vi "Logger.Stats.ListFiles.vi"(8 "error in (no error)":errorcluster) -> (0 "error out":errorcluster, 2 "Files":path[](array[path]))   [LabVIEW 2016]
uses:
  Global/ApplicationGlobal.vi
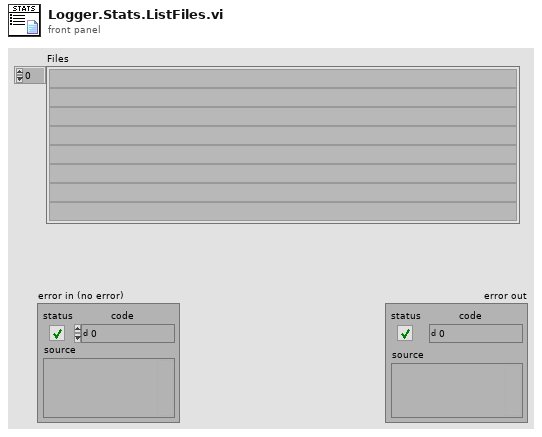
[diagram p1: front panel]
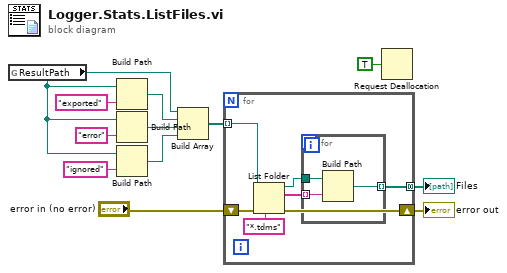
[diagram p0: block diagram]
diagram:
  n1 = global read "ApplicationGlobal.vi" "ResultPath"() -> (w5:path)
  n2 = Build Path(base path=w5, name or relative path="exported") -> (appended path=w9:path)
  n3 = Build Path(base path=w5, name or relative path="error") -> (appended path=w6:path)
  n4 = Build Path(base path=w5, name or relative path="ignored") -> (appended path=w8:path)
  n5 = Build Array(w5, w9, w6, w8) -> (w7:path[])
  n6 = for {
    tunnel: w7 -> [w18] mode=indexing
    tunnel: [w14] -> w1 mode=concatenating
    shift-right: [w13] -> w2
    shift-left: "error in (no error)" -> [w19]
    n7 = List Folder(path=w18, pattern="*.tdms", error in=w19) -> (path out=w16:path, filenames=w17:string[], error out=w13:errorcluster)  [unwired: 1 in, 1 out]
    n8 = for {
      tunnel: w17 -> [w22] mode=indexing
      tunnel: w16 -> [w21]
      tunnel: [w20] -> w14 mode=indexing
      n9 = Build Path(base path=w21, name or relative path=w22) -> (appended path=w20:path)
    }
  }
  "error out" <- w2
  "Files" <- w1
  n10 = Request Deallocation(TRUE ("flag")) -> ()
